vi "Untitled 3.vi"() -> ()   [LabVIEW 2019]
uses:
  <vilib>/userDefined/High Color/IMAQdx.ctl
  <vilib>/vision/driver/NI_Vision_Acquisition_Software.lvlib
panel:
  out "Image":T1(plugin-control)
  out "Numeric":dbl
  in  "stop":bool
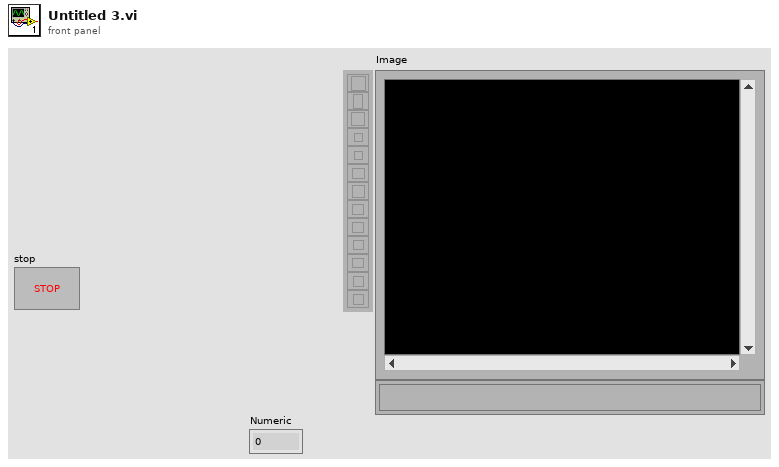
[diagram p1: front panel]
types:
  T1 = typedef "IMAQ Image.ctl" = refnum<image>
  T2 = typedef "IMAQdx.ctl" = refnum<k21>
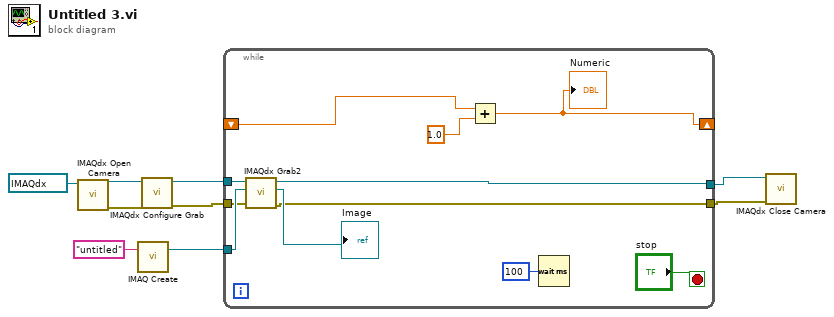
[diagram p0: block diagram]
diagram:
  n1 = call <vilib>:"IMAQdx Open Camera.vi"("Session In"=T2 "cam1") -> ("error out"=w7:errorcluster, "Session Out"=w8:T2)  [unwired: 9 in]
  n2 = call "IMAQ Create"("Image Name"="untitled") -> ("New Image"=w6:T1)  [unwired: 4 in, 1 out]
  n3 = call <vilib>:"IMAQdx Configure Grab.vi"("error in"=w7, "Session In"=w8) -> ("error out"=w3:errorcluster, "Session Out"=w4:T2)  [unwired: 8 in]
  n4 = while {
    tunnel: w6 -> [w20]
    shift-right: [w16] -> _
    shift-left: _ -> [w17]
    tunnel: w4 -> [w14]
    tunnel: w3 -> [w13]
    tunnel: [w12] -> w2
    tunnel: [w11] -> w1
    stop <- "stop" stop-if-true
    n5 = call <vilib>:"IMAQdx Grab2.vi"("error in"=w13, "Image In"=w20, "Session In"=w14) -> ("error out"=w12:errorcluster, "Image Out"=→"Image":T1, "Session Out"=w11:T2)  [unwired: 5 in, 1 out]
    n6 = Add(x=w17, y=1.0) -> (x+y=w16:dbl)
    "Numeric" <- w16
    n7 = Wait (ms)(milliseconds to wait=u32 100) -> ()  [unwired: 1 out]
  }
  n8 = call <vilib>:"IMAQdx Close Camera.vi"("error in"=w2, "Session In"=w1) -> ()  [unwired: 9 in, 1 out]
